vi "AddLimit.vi"(8 "error in":errorcluster, 10 "Comparison":string, 11 "StringMeasure in":refnum<class "StringMeasure.lvclass">) -> (0 "error out":errorcluster, 2 "StringMeasureLimit":refnum<class "StringMeasureLimit.lvclass">, 3 "StringMeasure out":refnum<class "StringMeasure.lvclass">)   [LabVIEW 2021, in "ProligentXMLGenerator.lvlib" / "StringMeasure.lvclass"]
doc: "Add a MeasureLimit element.\n\nThe limit expression associated with the measure."
uses:
  StringMeasure.lvclass
  StringMeasure.lvclass/StringMeasure.ctl
  MeasureLimit/MeasureLimit.lvclass
  StringMeasureLimit/StringMeasureLimit.lvclass
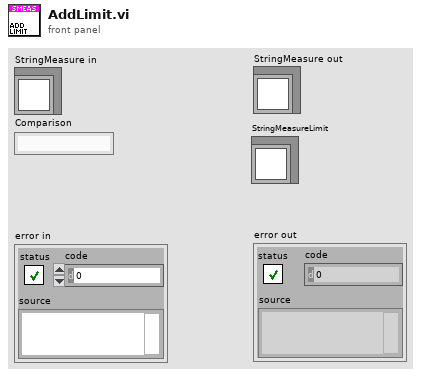
[diagram p1: front panel]
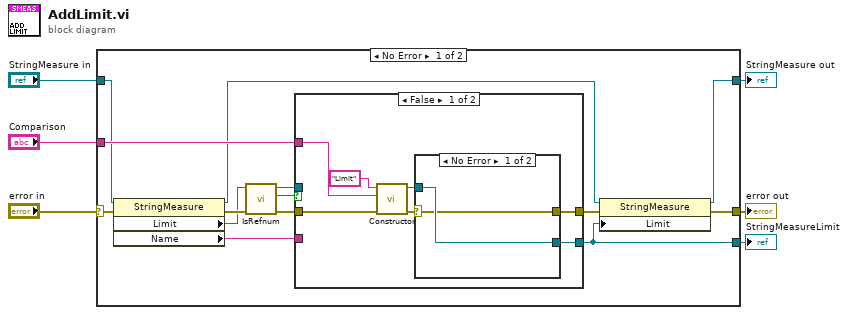
[diagram p0: block diagram]
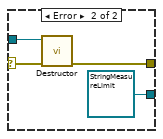
[diagram p2: hidden frame]
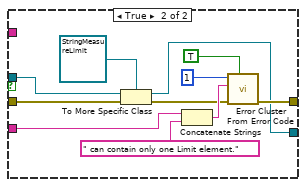
[diagram p3: hidden frame]
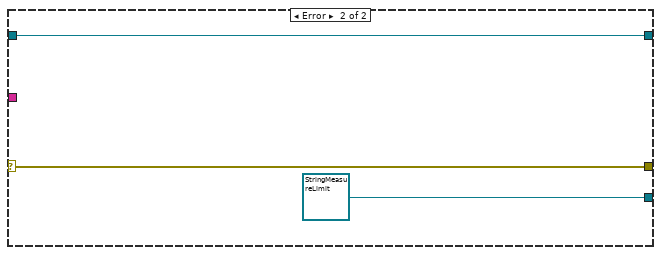
[diagram p4: hidden frame]
diagram:
  n1 = case shown="No Error" "error in" {
    selector: "error in" -> [w19 w46]
    tunnel: [w11 refnum<class "StringMeasureLimit.lvclass"> refnum ("ProligentResultProcessor:StringMeasureLimit")] -> w2
    tunnel: [w13 w46] -> w5
    tunnel: "StringMeasure in" -> [w10 w47]
    tunnel: [w12 w47] -> w3
    tunnel: "Comparison" -> [w14 _]
    frame No Error {
      n2 = property class="StringMeasure"(reference=w10, error in=w19) -> (reference out=w9:refnum<class "StringMeasure.lvclass">, error out=w18:errorcluster, "Limit"=w8:refnum<class "MeasureLimit.lvclass">, "Name"=w17:string)
      n3 = call "IsRefnum.vi"("error in"=w18, "MeasureLimit in"=w8) -> ("error out"=w16:errorcluster, "IsRefnum"=w15:bool, "MeasureLimit out"=w7:refnum<class "MeasureLimit.lvclass">)  [unwired: 7 in]
      n4 = case shown="False" w15 {
        tunnel: w16 -> [w23 w37]
        tunnel: [w27 w40] -> w20
        tunnel: [w26 w35] -> w11
        tunnel: w17 -> [_ w39]
        tunnel: w14 -> [w25 _]
        tunnel: w7 -> [_ w38]
        frame False {
          n5 = call "Constructor.vi"("error in"=w23, "Comparison"=w25, "Name"="Limit") -> ("error out"=w22:errorcluster, "StringMeasureLimit"=w21:refnum<class "StringMeasureLimit.lvclass">)  [unwired: 7 in]
          n6 = case shown="No Error" w22 {
            selector: w22 -> [w28 w33]
            tunnel: w21 -> [w29 w31]
            tunnel: [w28 w32] -> w27
            tunnel: [w29 refnum<class "StringMeasureLimit.lvclass"> refnum ("ProligentResultProcessor:StringMeasureLimit")] -> w26
            frame No Error {
            }
            frame Error {
              n7 = call "Destructor.vi"("error in"=w33, "StringMeasureLimit"=w31) -> ("error out"=w32:errorcluster)  [unwired: 9 in]
            }
          }
        }
        frame True {
          n8 = To More Specific Class(target class=refnum<class "StringMeasureLimit.lvclass"> refnum ("ProligentResultProcessor:StringMeasureLimit"), reference=w38, error in=w37) -> (specific class reference=w35:refnum<class "StringMeasureLimit.lvclass">, error out=w36:errorcluster)
          n9 = Concatenate Strings(w39, " can contain only one Limit element." ("string")) -> (w44:string)
          n10 = call <vilib>:"Error Cluster From Error Code.vi"("show call chain? (False)"=TRUE, "error in (no error)"=w36, "error message (\"\")"=w44, "error code (0)"=1) -> ("error out"=w40:errorcluster)  [unwired: 5 in]
        }
      }
      n11 = property class="StringMeasure"(reference=w9, error in=w20, "Limit"=w11) -> (reference out=w12:refnum<class "StringMeasure.lvclass">, error out=w13:errorcluster)
    }
    frame Error {
    }
  }
  "error out" <- w5
  "StringMeasure out" <- w3
  "StringMeasureLimit" <- w2
